vi "Send Message.vi"(4 "timeout in ms (100)":i32=100, 8 "error in (no error)":errorcluster, 9 "Message ID":u32, 10 "Message":T1, 11 "RemoteControl in":refnum<class "RemoteControl.lvclass">) -> (0 "error out":errorcluster, 3 "RemoteControl out":refnum<class "RemoteControl.lvclass">)   [LabVIEW 2016, in "RemoteControl.lvclass"]
uses:
  RemoteControl.lvclass
  Typedefs/Message--Cluster.ctl
  RemoteControlGlobal.vi
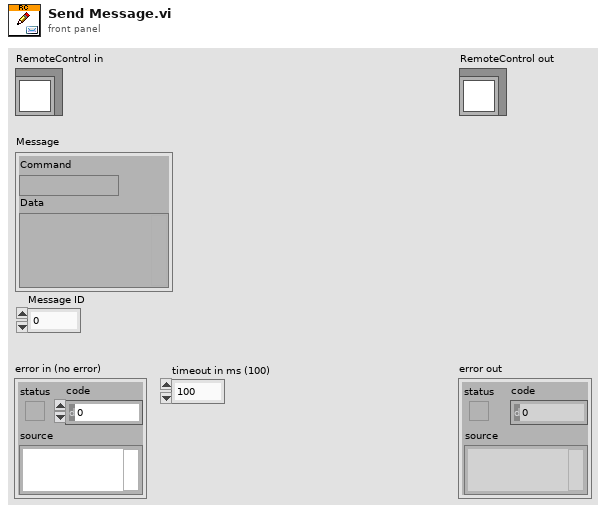
[diagram p1: front panel]
types:
  T1 = typedef "RemoteControl.lvclass/Message--Cluster.ctl" = cluster{"Command":string, "Data":variant}
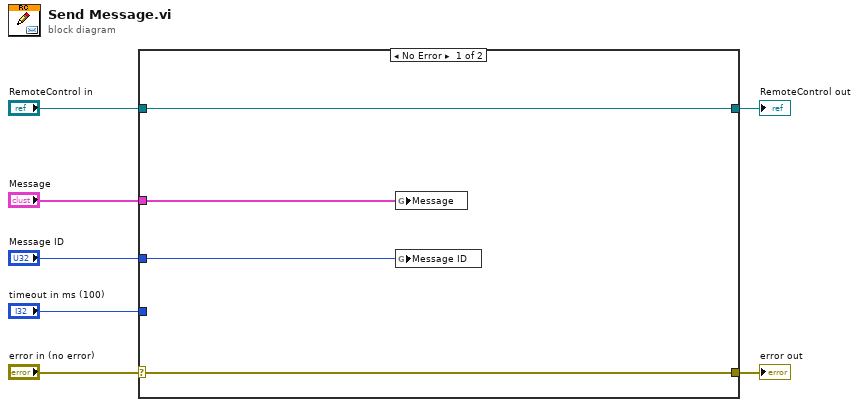
[diagram p0: block diagram]
diagram:
  n1 = case shown="No Error" "error in (no error)" {
    selector: "error in (no error)" -> [w10 w13]
    tunnel: [w10 w13] -> w6
    tunnel: [w11 w12] -> w4
    tunnel: "RemoteControl in" -> [w11 w12]
    tunnel: "Message" -> [w8 _]
    tunnel: "Message ID" -> [w9 _]
    tunnel: "timeout in ms (100)" -> [_ _]
    frame No Error {
      n2 = global write "RemoteControlGlobal.vi" "Message"(w8) -> ()
      n3 = global write "RemoteControlGlobal.vi" "Message ID"(w9) -> ()
    }
    frame Error {
    }
  }
  "error out" <- w6
  "RemoteControl out" <- w4
